vi "bitstream_to_32bitv2.vi"(8 "error in (no error)":errorcluster, 10 "JPG Size":i32[](array[numeric])=[0, 0], 11 "Bitstream Input":u8[](array[numeric])) -> (0 "error out":errorcluster, 1 "2D JPG Array":u32[][](array[numeric]))   [LabVIEW 2013]
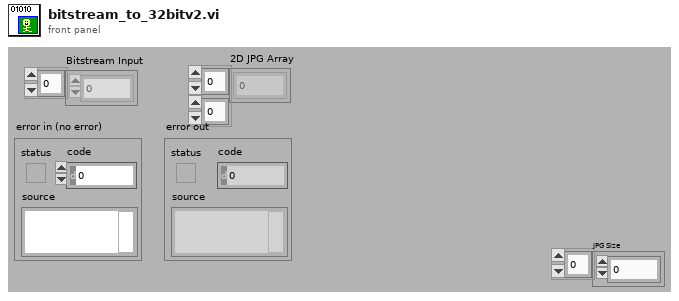
[diagram p1: front panel]
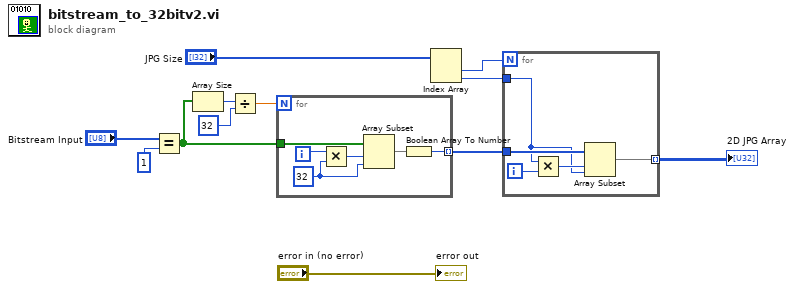
[diagram p0: block diagram]
diagram:
  n1 = Equal?(x="Bitstream Input", y=u8 1) -> (x = y?=w7:bool[])
  n2 = Array Size(array=w7) -> (size(s)=w8:i32)
  n3 = Divide(x=w8, y=32) -> (x/y=w10:dbl)
  n4 = for {
    N: w10 -> [_]
    tunnel: w7 -> [w18]
    tunnel: [w13] -> w11 mode=indexing
    i -> [w15]
    w16 = 32 ("y")
    n5 = Multiply(x=w15, y=w16) -> (x*y=w17:i32)
    n6 = Array Subset(array=w18, index=w17, length=w16) -> (w14:bool[])
    n7 = Boolean Array To Number(Boolean array=w14) -> (number=w13:u32)
  }
  n8 = Index Array(array="JPG Size") -> (element #1=w3:i32, element #2=w2:i32)  [unwired: 2 in]
  n9 = for {
    N: w3 -> [_]
    tunnel: w11 -> [w23]
    tunnel: [w20] -> w12 mode=indexing
    tunnel: w2 -> [w19]
    i -> [w22]
    n10 = Multiply(x=w19, y=w22) -> (x*y=w21:i32)
    n11 = Array Subset(array=w23, index=w21, length=w19) -> (w20:u32[])
  }
  "2D JPG Array" <- w12
  "error out" <- "error in (no error)"
